vi "2100_Update_Single_Register_Bits.vi"(7 "Reg_Address_Data":T1={"Address"=81, "Data"=0} {"Address" format="%.0x"}, 8 "Error In":errorcluster, 9 "Length":u8=5, 10 "LSB":u8, 11 "Master_Register_Data_Array_In":T2 {"Address" format="%.0x"}) -> (0 "Error Out":errorcluster, 2 "Single_Reg_Address_Data Out":T1={"Address"=81, "Data"=0} {"Address" format="%.0x"}, 3 "Master_Register_Data_Array_Out":T2 {"Address" format="%.0x"})   [LabVIEW 2013]
uses:
  Controls/Master_Reg_Data_Array.ctl
  Controls/Reg_Address_Data.ctl
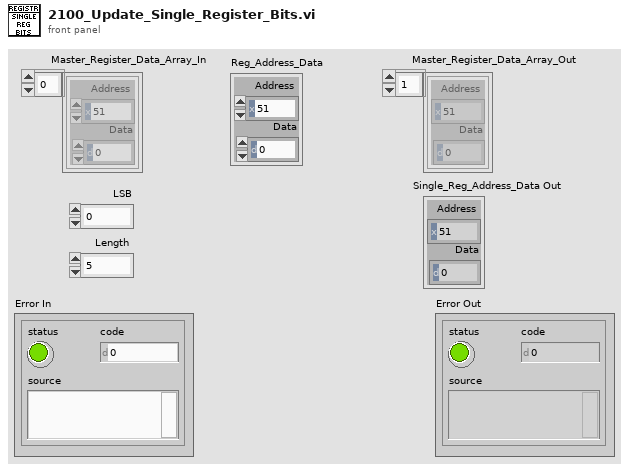
[diagram p1: front panel]
types:
  T1 = typedef "Reg_Address_Data.ctl" = cluster{"Address":u8, "Data":u8}
  T2 = typedef "Master_Reg_Data_Array.ctl" = T1[]
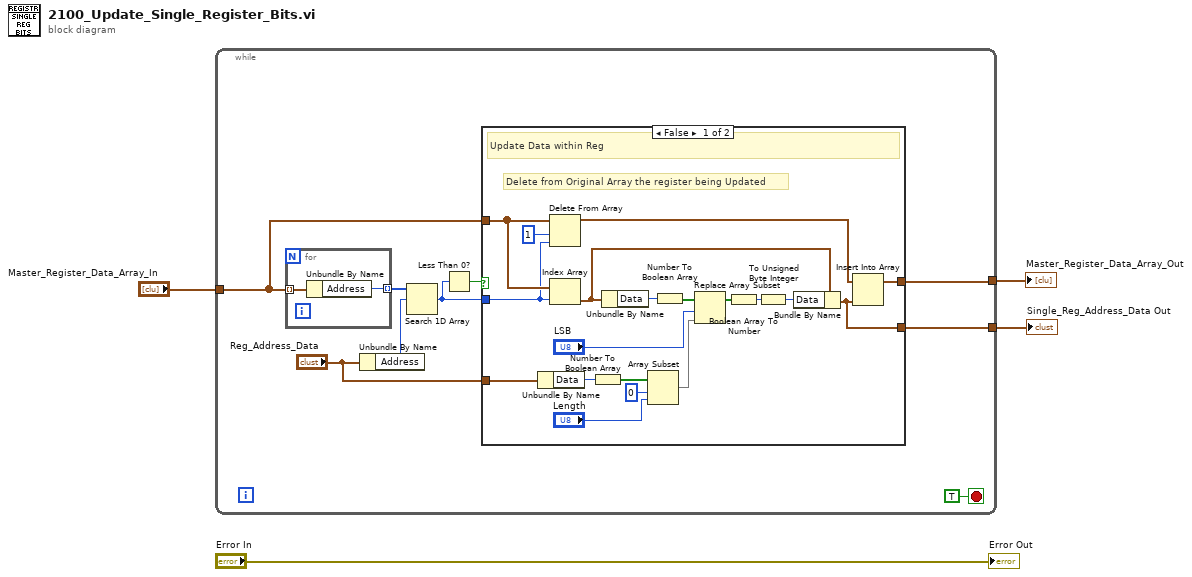
[diagram p0: block diagram]
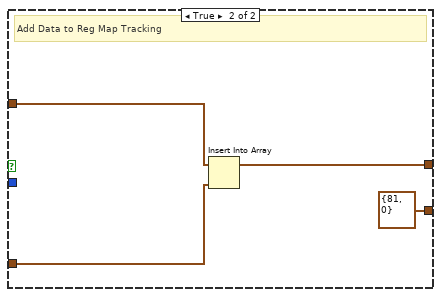
[diagram p2: hidden frame]
diagram:
  n1 = while {
    tunnel: [w12] -> w4
    tunnel: "Master_Register_Data_Array_In" -> [w11]
    tunnel: [w5] -> w1
    stop <- TRUE stop-if-true
    n2 = for {
      tunnel: w11 -> [w38] mode=indexing
      tunnel: [w37] -> w10 mode=indexing
      n3 = Unbundle By Name(w38) -> ("Address"=w37:u8)
    }
    n4 = Unbundle By Name("Reg_Address_Data") -> ("Address"=w9:u8)
    n5 = Search 1D Array(1D array=w10, element=w9) -> (index of element=w8:i32)  [unwired: 1 in]
    n6 = Less Than 0?(x=w8) -> (x < 0?=w7:bool)
    n7 = case shown="False" w7 {
      tunnel: [w21 w35] -> w12
      tunnel: w11 -> [w20 w36]
      tunnel: w8 -> [w19 _]
      tunnel: "Reg_Address_Data" -> [w16 w34]
      tunnel: [w14 T1 {"Address"=81, "Data"=0} ("Reg_Address_Data 2")] -> w5
      frame False {
        # "Delete from Original Array the register being Updated"
        # "Update Data within Reg"
        n8 = Unbundle By Name(w16) -> ("Data"=w15:u8)
        n9 = Delete From Array(array=w20, length=1, index=w19) -> (array with subset deleted=w22:T2)  [unwired: 1 out]
        n10 = Index Array(array=w20, index=w19) -> (element=w26:T1)
        n11 = Number To Boolean Array(number=w15) -> (Boolean array=w30:bool[])
        n12 = Unbundle By Name(w26) -> ("Data"=w25:u8)
        n13 = Array Subset(array=w30, index=u8 0, length="Length") -> (w28:bool[])
        n14 = Number To Boolean Array(number=w25) -> (Boolean array=w31:bool[])
        n15 = Replace Array Subset(array=w31, new element=w28, index="LSB") -> (w29:bool[])
        n16 = Boolean Array To Number(Boolean array=w29) -> (number=w32:u32)
        n17 = To Unsigned Byte Integer(number=w32) -> (unsigned 8bit integer=w24:u8)
        n18 = Bundle By Name(cluster=w26, "Data"=w24) -> (w14:T1)
        n19 = Insert Into Array(array=w22, new element=w14) -> (w21:T2)  [unwired: 1 in]
      }
      frame True {
        # "Add Data to Reg Map Tracking"
        n20 = Insert Into Array(array=w36, new element=w34) -> (w35:T2)  [unwired: 1 in]
      }
    }
  }
  "Master_Register_Data_Array_Out" <- w4
  "Single_Reg_Address_Data Out" <- w1
  "Error Out" <- "Error In"
